vi "average_v1.vi"(7 "Numeric 4":fxp<+/-,24,1>, 8 "Numeric 3":fxp<+/-,24,1>, 9 "Numeric 2":fxp<+/-,24,1>, 10 "Numeric":fxp<+/-,24,1>) -> (2 "rms2":fxp<+/-,24,1> format="%.24g", 3 "mean":fxp<+/-,31,3>)   [LabVIEW 2014]
uses:
  <vilib>/rvi/Emulation/niFpgaProcessEmulError.vi
  <vilib>/rvi/FXPMathLib/FxpMul/XNode/nifxpmath_Multiplier.xnode
  <vilib>/rvi/FXPMathLib/FxpAdd/XNode/nifxpmath_Add.xnode
  <vilib>/rvi/FXPMathLib/sim/FxpSim.dll
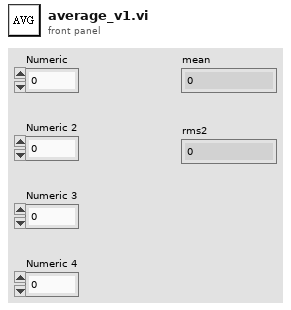
[diagram p1: front panel]
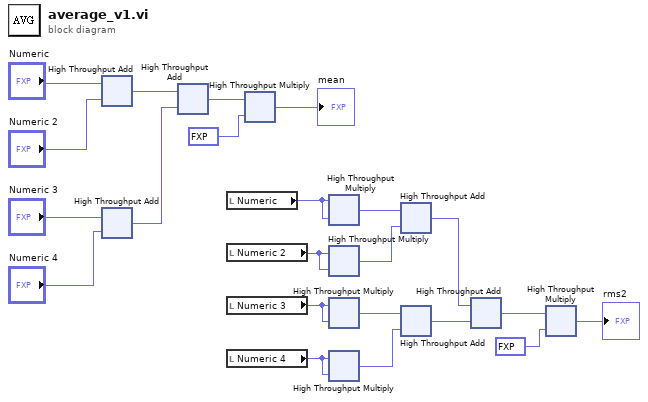
[diagram p0: block diagram]
diagram:
  n1 = xnode "High Throughput Add"("x"="Numeric", "y"="Numeric 2") -> ("x+y"=w18:fxp<+/-,25,2>)
  n2 = xnode "High Throughput Add"("x"="Numeric 3", "y"="Numeric 4") -> ("x+y"=w17:fxp<+/-,25,2>)
  n3 = xnode "High Throughput Add"("x"=w18, "y"=w17) -> ("x+y"=w16:fxp<+/-,26,3>)
  n4 = local read "Numeric"() -> (w13:fxp<+/-,24,1>)
  n5 = local read "Numeric 2"() -> (w12:fxp<+/-,24,1>)
  n6 = local read "Numeric 3"() -> (w11:fxp<+/-,24,1>)
  n7 = local read "Numeric 4"() -> (w10:fxp<+/-,24,1>)
  n8 = xnode "High Throughput Multiply"("x"=w16, "y"=fxp<+/-,5,0> 0.25) -> ("x*y"=→"mean":fxp<+/-,31,3>)
  n9 = xnode "High Throughput Multiply"("x"=w13, "y"=w13) -> ("x*y"=w9:fxp<+/-,48,2>)
  n10 = xnode "High Throughput Multiply"("x"=w12, "y"=w12) -> ("x*y"=w8:fxp<+/-,48,2>)
  n11 = xnode "High Throughput Multiply"("x"=w11, "y"=w11) -> ("x*y"=w7:fxp<+/-,48,2>)
  n12 = xnode "High Throughput Multiply"("x"=w10, "y"=w10) -> ("x*y"=w6:fxp<+/-,48,2>)
  n13 = xnode "High Throughput Add"("x"=w9, "y"=w8) -> ("x+y"=w4:fxp<+/-,49,3>)
  n14 = xnode "High Throughput Add"("x"=w7, "y"=w6) -> ("x+y"=w5:fxp<+/-,49,3>)
  n15 = xnode "High Throughput Add"("x"=w4, "y"=w5) -> ("x+y"=w3:fxp<+/-,50,4>)
  n16 = xnode "High Throughput Multiply"("x"=w3, "y"=fxp<+/-,5,0> 0.25) -> ("x*y"=→"rms2":fxp<+/-,24,1>)
